vi "Confirm Action.vi"(11 "Confirm?":bool) -> (3 "T button?":bool)   [LabVIEW 2012, in "Configuration Grandmaster.lvlib" / "Cfg Grandmaster.lvclass"]
uses:
  Cfg Grandmaster.lvclass
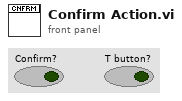
[diagram p1: front panel]
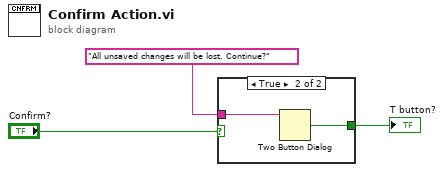
[diagram p0: block diagram]
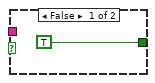
[diagram p2: hidden frame]
diagram:
  n1 = case shown="True" "Confirm?" {
    tunnel: [TRUE w6] -> w3
    tunnel: "All unsaved changes will be lost. Continue?" -> [_ w5]
    frame False {
    }
    frame True {
      n2 = Two Button Dialog(message=w5) -> (T button?=w6:bool)  [unwired: 2 in]
    }
  }
  "T button?" <- w3
